vi "AngeloRTV Initialize Image Array.vi"(2 "Error_In":i16, 4 "PortNo":u16) -> (0 "Error_Out":i16, 1 "Initialized Array":T1)   [LabVIEW 2012]
panel:
  in  "Initialized Array ctl.":T1
  in  "vi name":string="AngeloRTV Initialize Image Array.vi"
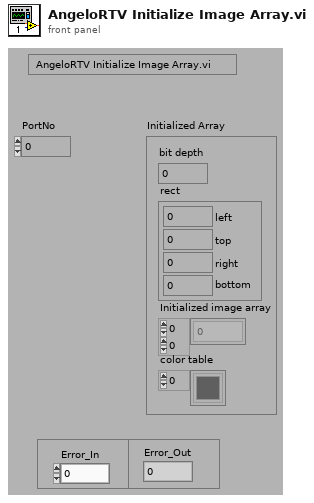
[diagram p1: front panel]
types:
  T1 = cluster{"bit depth":u8, "rect":cluster{"left":i16, "top":i16, "right":i16, "bottom":i16}, "Initialized image array":u8[][], "color table":u32[]}
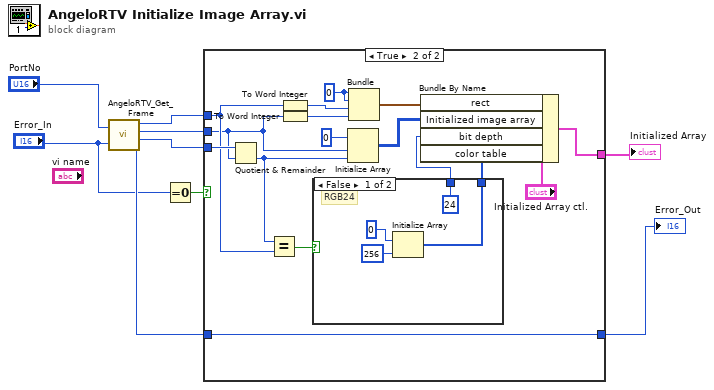
[diagram p0: block diagram]
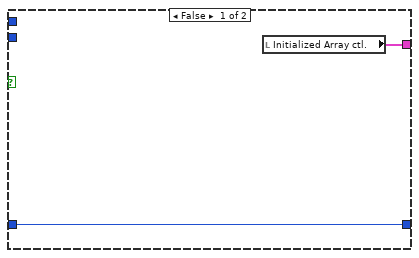
[diagram p2: hidden frame]
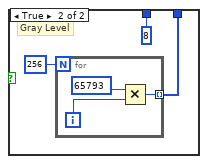
[diagram p3: hidden frame]
diagram:
  n1 = call "AngeloRTV_Get_Frame.vi"("Error_In"="Error_In", "PortNo"="PortNo") -> ("Error_Out"=w4:i16, "Szie_Byte"=w8:u32, "Height"=w7:u32, "Width"=w6:u32)  [unwired: 1 out]
  n2 = Equal To 0?(x="Error_In") -> (x = 0?=w2:bool)
  n3 = case shown="True" w2 {
    tunnel: w8 -> [_ w27]
    tunnel: w7 -> [_ w19]
    tunnel: w6 -> [_ w20]
    tunnel: [w10 w24] -> w5
    tunnel: w4 -> [w11 w22]
    tunnel: [w11 w22] -> w3
    frame False {
      n4 = local read "Initialized Array ctl."() -> (w10:T1)
    }
    frame True {
      w16 = i16 0
      n5 = Quotient & Remainder(x=w27, y=w19) -> (floor(x/y)=w25:u32)  [unwired: 1 out]
      n6 = Equal?(x=w25, y=w20) -> (x = y?=w23:bool)
      n7 = To Word Integer(number=w20) -> (16bit integer=w18:i16)
      n8 = To Word Integer(number=w19) -> (16bit integer=w17:i16)
      n9 = case shown="False" w23 {
        tunnel: [w29 w33] -> w13
        tunnel: [u8 24 u8 8] -> w12
        frame False {
          # "RGB24"
          n10 = Initialize Array(u32 0 ("Element Data"), 256 ("Dimension Size")) -> (w29:u32[])
        }
        frame True {
          # "Gray Level"
          n11 = for {
            N: 256 -> [_]
            tunnel: [w35] -> w33 mode=indexing
            i -> [w37]
            n12 = Multiply(x=u32 65793, y=w37) -> (x*y=w35:u32)
          }
        }
      }
      n13 = Initialize Array(u8 0 ("Element Data"), w19, w25) -> (w14:u8[][])
      n14 = Bundle(w16, w16, w18, w17) -> (w15:cluster{i16, i16, i16, i16})  [unwired: 1 in]
      n15 = Bundle By Name(cluster="Initialized Array ctl.", "rect"=w15, "Initialized image array"=w14, "bit depth"=w12, "color table"=w13) -> (w24:T1)
    }
  }
  "Initialized Array" <- w5
  "Error_Out" <- w3
